vi "RRTPlan.vi"(5 "Parameters.lvclass":refnum<class "Parameters.lvclass">, 6 "Line?":bool, 7 "Volta ao redor\nda área?":bool, 8 "Initial Pos x,y":dbl[](array[numeric]), 9 "Dest x,y":dbl[](array[numeric]), 10 "IA State":T1={"our_robots"=[], "enemy_robots"=[], "balls"=[], "geometry"={"line_width"=0, "field_length"=0, "field_width"=0, "boundary_width"=0, "referee_width"=0, "goal_width"=0, "goal_depth"=0, "goal_wall_width"=0, "center_circle_radius"=0, "defense_radius"=0, "defense_stretch"=0, "free_kick_from_defense_dist"=0, "penalty_spot_from_field_line_dist"=0, "penalty_line_from_spot_dist"=0}, "IA Judge"={"stage"="", "command"="", "our_goalie_id"=0.0, "enemy_goalie_id"=0.0, "command enum"=enum."Halt", "Time"=enum."Azul"}, "Received Timestamp"=timestamp(0 s since 1904-01-01), "Events"={"Touch"=FALSE, "Ball out"=FALSE, "id touch"=0.0, "Ball out of \nVision"=FALSE, "Ball inside \nGoalie area"=FALSE, "Robot not responding"=FALSE, "Robots responding status"=[1.0, 1.0, 1.0, 1.0, 1.0, 1.0], "Enemy Ball \nPossession"=FALSE, "Pass State"=FALSE, "id end of pass"=0.0, "Kick"=FALSE, "Id ini Possession"=0.0, "Ball Possesion"=FALSE, "Id Possesion"=0.0, "Direct Kick"=FALSE, "2nd Strk Ativo"=FALSE}}, 11 "Robot":T2={"id"=0, "function"=enum."Attacker", "x"=0.0, "y"=0.0, "orientation"=0.0, "v_tangent"=0.0, "v_normal"=0.0, "v_ang"=0.0, "kick_x"=0.0, "kick_z"=0.0, "dribble"=FALSE, "Timestamp"=timestamp(0 s since 1904-01-01), "estimatives"={"est_v_tangent"=0.0, "est_v_normal"=0.0, "est_vx"=0.0, "est_vy"=0.0, "Pos Robot Est"=[]}, "dest_x_kick"=0.0, "dest_y_kick"=0.0, "Gap Coord"=[], "States"=enum."GoToTangent", "Path "=[], "Path  Smooth"=[], "Dest"=[], "vx_desired"=0.0, "vy_desired"=0.0, "slowBehavior"=FALSE, "VSSStates"=enum."Pass"}) -> (0 "Path":dbl[][](array[numeric]), 1 "Smooth Path":dbl[][](array[numeric]))   [LabVIEW 2020]
uses:
  Vision_class/Old vision/Controls/AI Robot.ctl
  Vision_class/Old vision/Controls/Functions Enum.ctl
  Vision_class/Old vision/Controls/AttackerStates.ctl
  Vision_class/Old vision/Controls/PathDests.ctl
  Vision_class/Old vision/Controls/PathDest.ctl
  Navigation/VSSNavigation/VSSAttackerStates.ctl
  Vision_class/Old vision/SSL Detection Frame Simple Estimator Cameras VelCmd Folder/Core/AI Input.ctl
  Vision_class/Old vision/SSL Detection Frame Simple Estimator Cameras VelCmd Folder/Core/AI Ball.ctl
  Vision_class/Old vision/SSL Detection Frame Simple Estimator Cameras VelCmd Folder/Core/Field Size.ctl
  Vision_class/Old vision/SSL Detection Frame Simple Estimator Cameras VelCmd Folder/Core/AI Judge.ctl
  Communication_class/Paths/MessageAI_State Folder/Intel/Command Enum.ctl
  Vision_class/Old vision/SSL Detection Frame Simple Estimator Cameras VelCmd Folder/Util/Events/Events.ctl
  Parameters_class/Parameters.lvclass
  Utilities_class/Utilities.lvclass
  Parameters_class/Parameters.lvclass/Parameters.ctl
  <vilib>/Analysis/_algsub.llb/Real Vector Norm.vi
  Parameters_class/Read Project.vi
  <vilib>/Analysis/NI_AALPro.lvlib
panel:
  in  "Path out":dbl[][](array[numeric])
  out "Path out 2":dbl[][](array[numeric])
  in  "WayPointProb":dbl=0.6 format="%#_13g"
  in  "GoalProb":dbl=0.1 format="%#_13g"
  in  "Step":dbl=80.0
  out "Goal":dbl[](array[numeric])
  out "Initial State":dbl[](array[numeric])
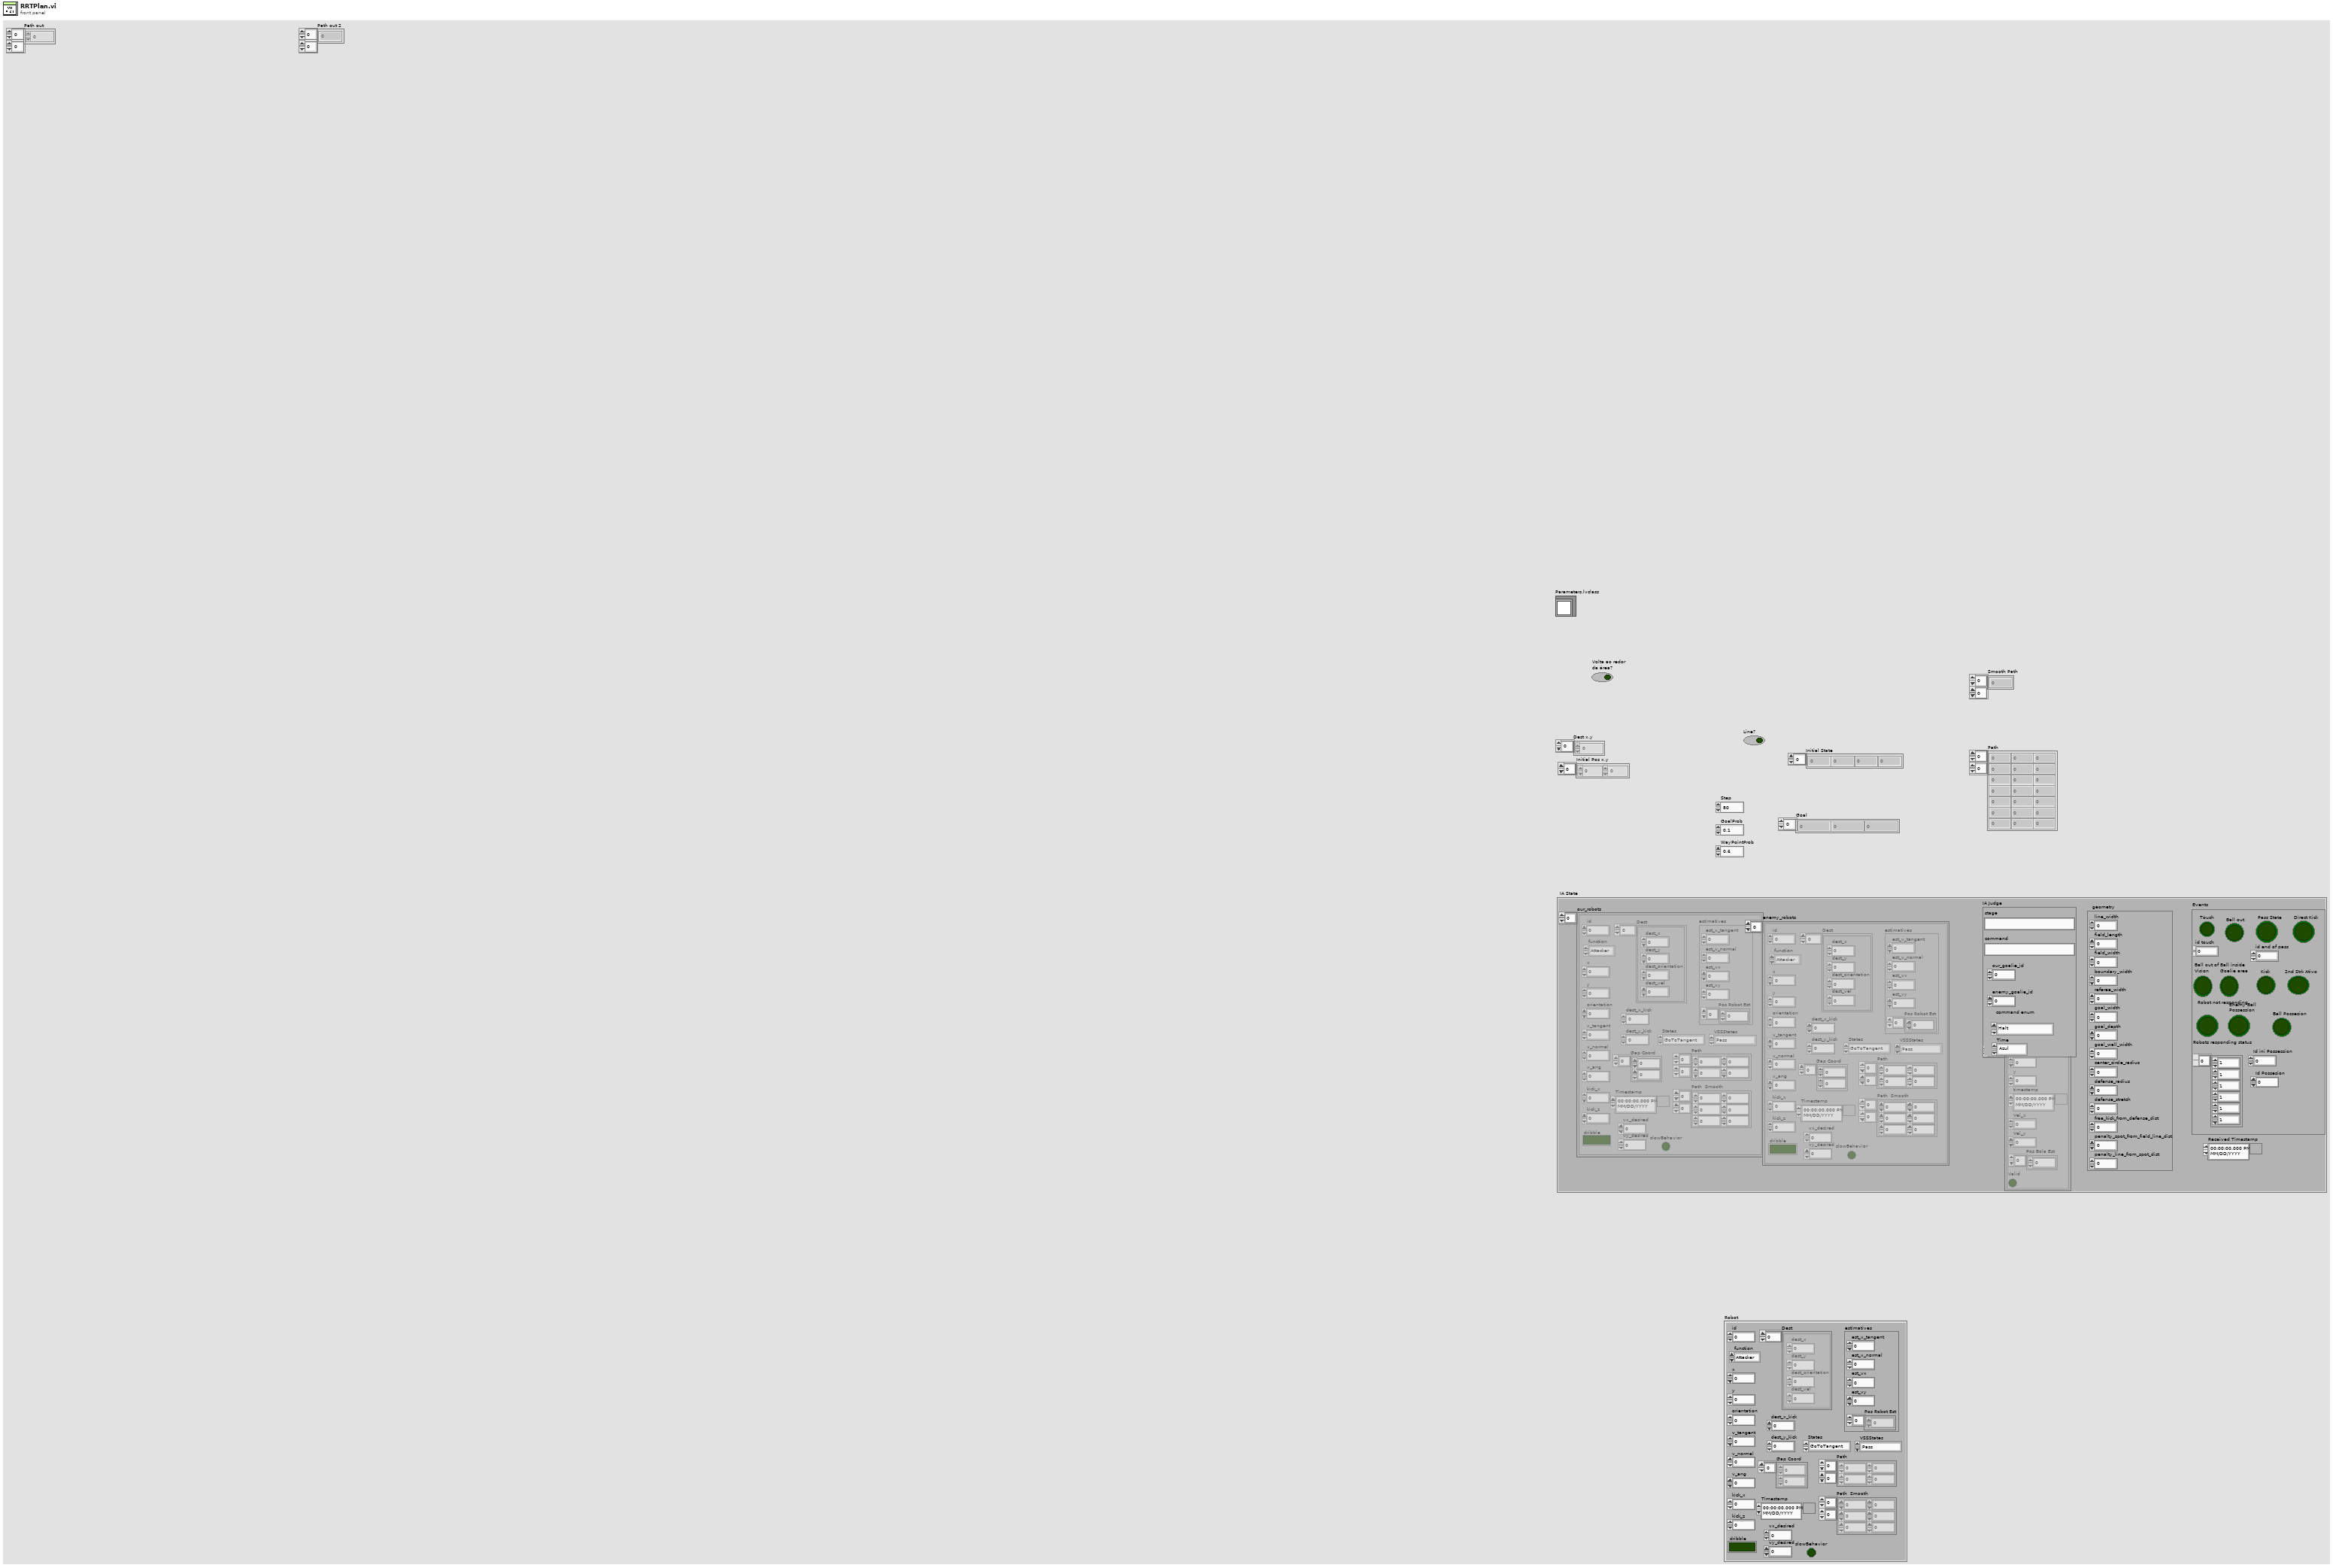
[diagram p1: front panel]
types:
  T1 = typedef "AI Input.ctl" = cluster{"our_robots":T2[], "enemy_robots":T2[], "balls":T8[], "geometry":T9, "IA Judge":T10, "Received Timestamp":timestamp, "Events":T12}
  T2 = typedef "AI Robot.ctl" = cluster{"id":u32, "function":T3, "x":dbl, "y":dbl, "orientation":dbl, "v_tangent":dbl, "v_normal":dbl, "v_ang":dbl, "kick_x":dbl, "kick_z":dbl, "dribble":bool, "Timestamp":timestamp, "estimatives":cluster{"est_v_tangent":dbl, "est_v_normal":dbl, "est_vx":dbl, "est_vy":dbl, "Pos Robot Est":dbl[]}, "dest_x_kick":dbl, "dest_y_kick":dbl, "Gap Coord":dbl[], "States":T4, "Path ":dbl[][], "Path  Smooth":dbl[][], "Dest":T5, "vx_desired":dbl, "vy_desired":dbl, "slowBehavior":bool, "VSSStates":T7}
  T3 = typedef "Functions Enum.ctl" = enum16{"2nd Striker", "Attacker", "Goalie", "Defender", "Striker", "Goto 0", "Dummy", "Kicker", "ZigZag 0", "ZigZag 1", "ZigZag 2", "ZigZag 3", "ZigZag 4", "ZigZag 5", "ZigZag 6", "ZigZag 7", "ZigZag 8", ""}
  T4 = typedef "AttackerStates.ctl" = enum16{"Pass", "GoToTangent", "BallGetting", "GoToKick", ""}
  T5 = typedef "PathDests.ctl" = T6[]
  T6 = typedef "PathDest.ctl" = cluster{"dest_x":dbl, "dest_y":dbl, "dest_orientation":dbl, "dest_vel":dbl}
  T7 = typedef "VSSAttackerStates.ctl" = enum16{"Pass", "GoToTangent", "BallGetting", "GoToKick", "Rotate anti-clockwise", "Rotate Clockwise", ""}
  T8 = typedef "AI Ball.ctl" = cluster{"x":dbl, "y":dbl, "timestamp":timestamp, "Vel_x":dbl, "Vel_y":dbl, "Pos Bola Est":dbl[], "Valid":bool}
  T9 = typedef "Field Size.ctl" = cluster{"line_width":u32, "field_length":u32, "field_width":u32, "boundary_width":u32, "referee_width":u32, "goal_width":u32, "goal_depth":u32, "goal_wall_width":u32, "center_circle_radius":u32, "defense_radius":u32, "defense_stretch":u32, "free_kick_from_defense_dist":u32, "penalty_spot_from_field_line_dist":u32, "penalty_line_from_spot_dist":u32}
  T10 = typedef "AI Judge.ctl" = cluster{"stage":string, "command":string, "our_goalie_id":dbl, "enemy_goalie_id":dbl, "command enum":T11, "Time":enum16{"Azul", "Amarelo"}}
  T11 = typedef "Command Enum.ctl" = enum16{"Halt", "Stop", "Force Start", "PKA Normal Start", "Prepare Kickoff Ally", "PKE Normal Start", "Prepare Kickoff Enemy", "Prepare Penalty Ally", "PPA Normal Start", "Prepare Penalty Enemy", "PPE Normal Start", "Direct Free Enemy", "Direct Free Ally", "Indirect Free Enemy", "Indirect Free Ally", "Timeout Enemy", "Timeout Ally", "Goal Enemy", "Goal Ally", "Ball Placement Enemy", "Ball Placement Ally", "Normal Half Time", "Extra Time Break", "Extra Half Time", "None", "Post Game"}
  T12 = typedef "Events.ctl" = cluster{"Touch":bool, "Ball out":bool, "id touch":dbl, "Ball out of \nVision":bool, "Ball inside \nGoalie area":bool, "Robot not responding":bool, "Robots responding status":dbl[], "Enemy Ball \nPossession":bool, "Pass State":bool, "id end of pass":dbl, "Kick":bool, "Id ini Possession":dbl, "Ball Possesion":bool, "Id Possesion":dbl, "Direct Kick":bool, "2nd Strk Ativo":bool}
  T13 = typedef "Project.ctl" = enum16{"SSL", "VSS"}
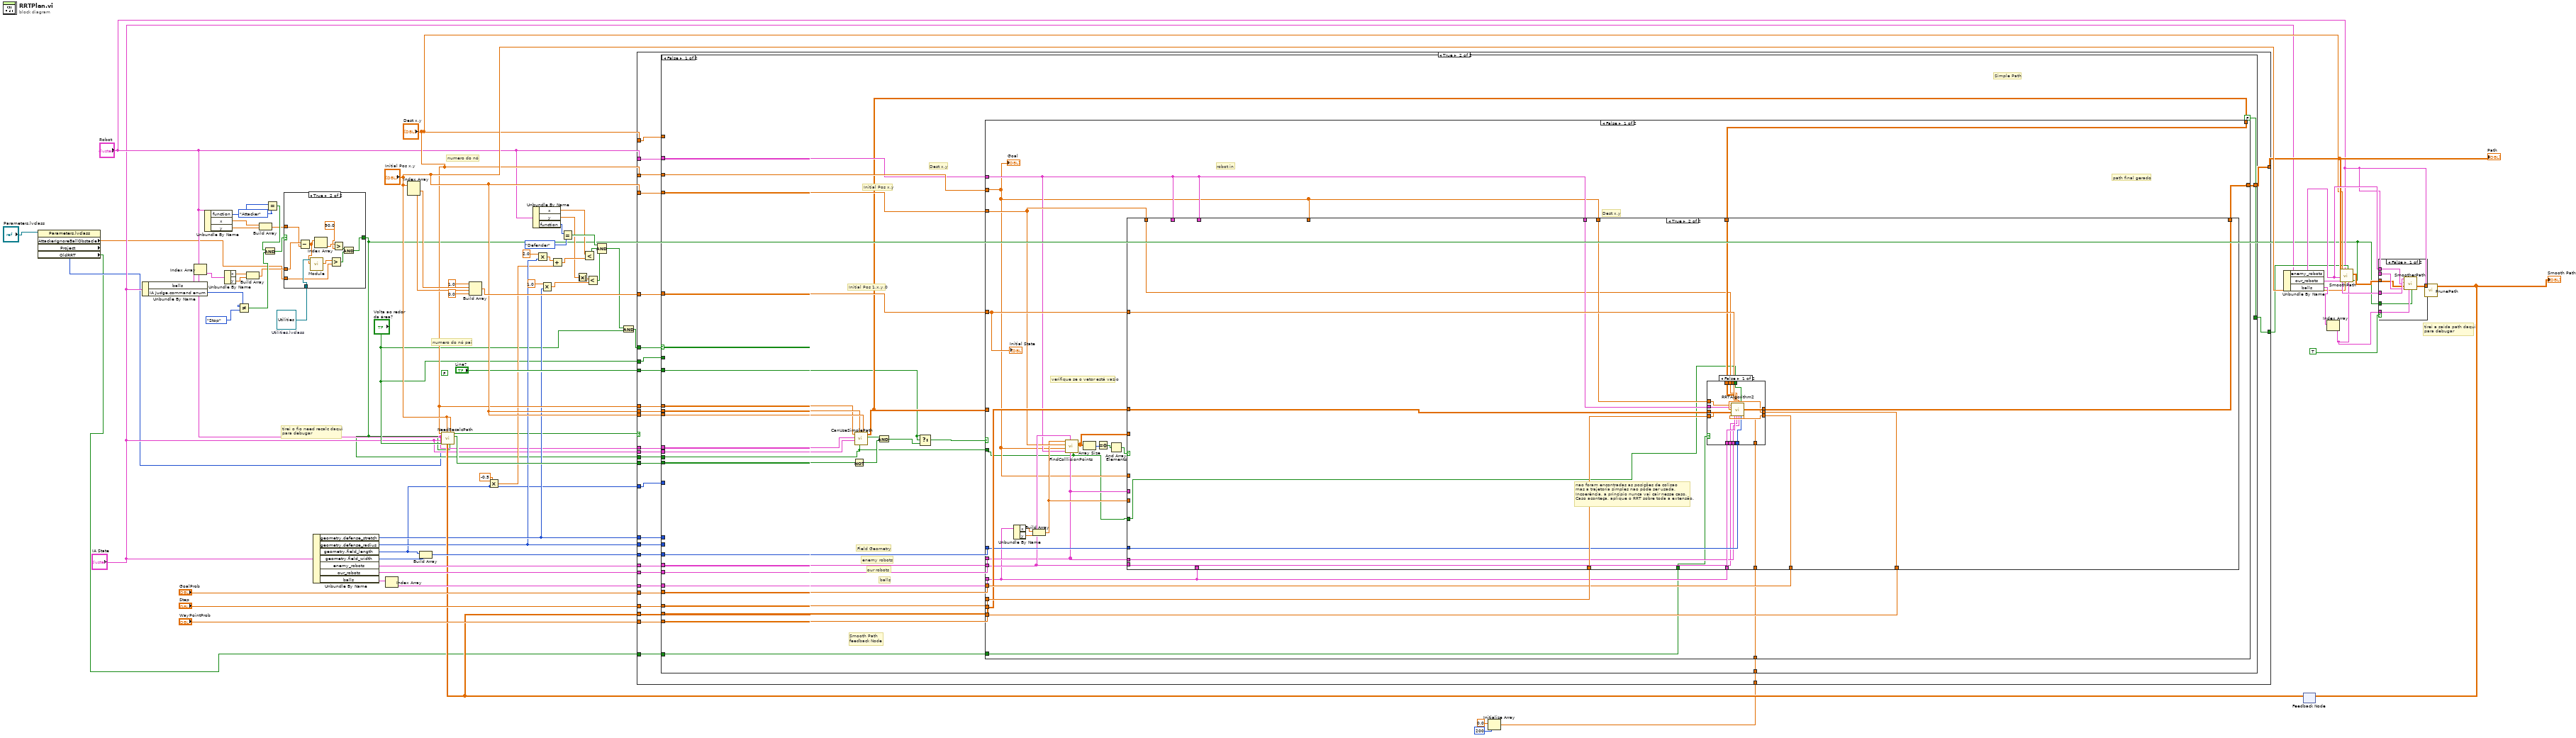
[diagram p0: block diagram]
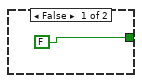
[diagram p2: hidden frame]
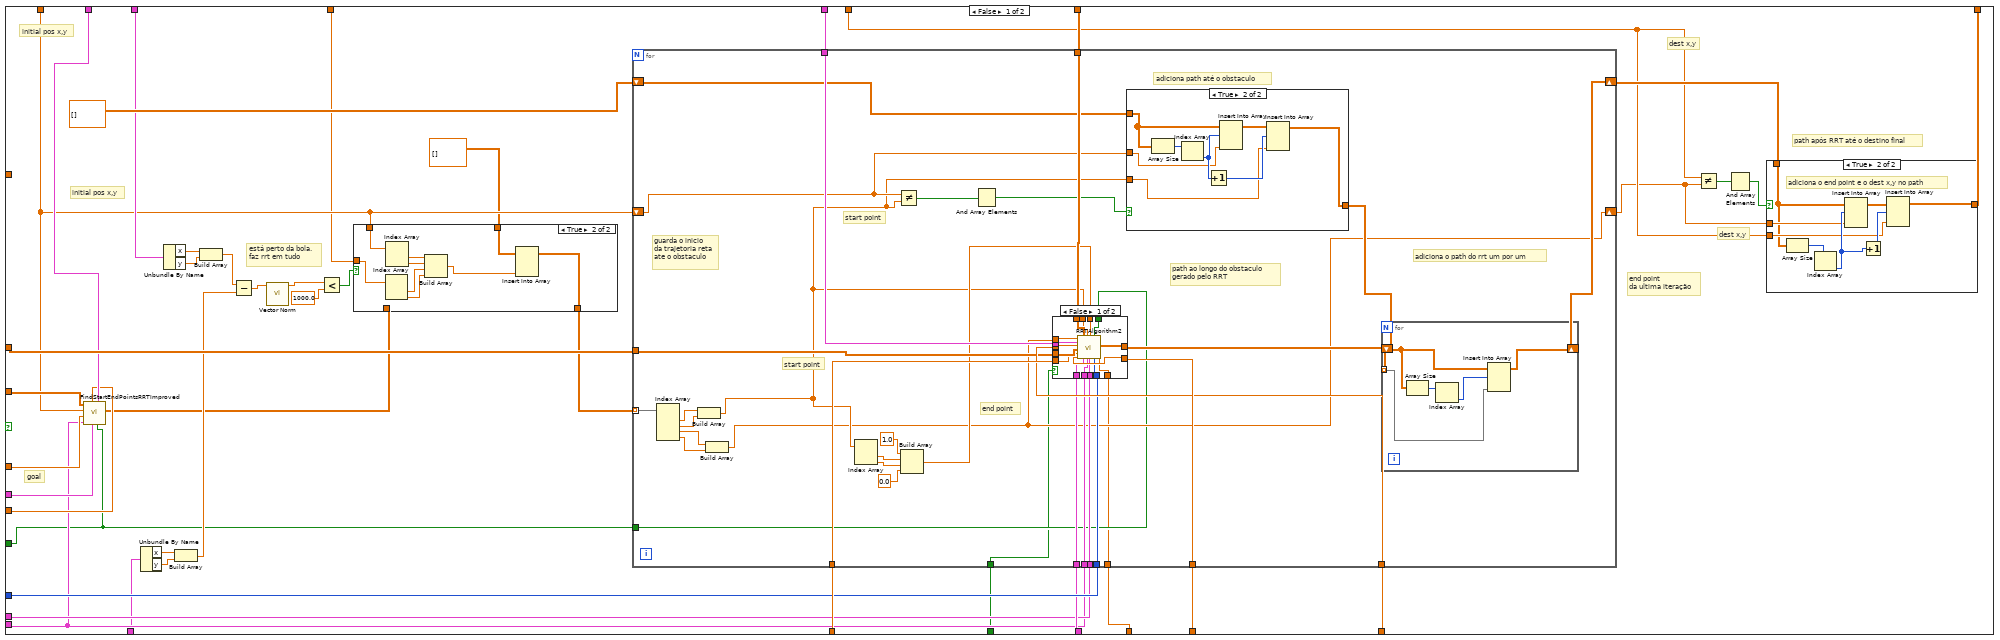
[diagram p4: hidden frame]
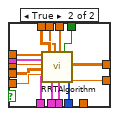
[diagram p7: hidden frame]
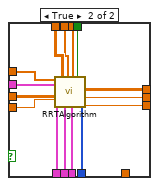
[diagram p9: hidden frame]
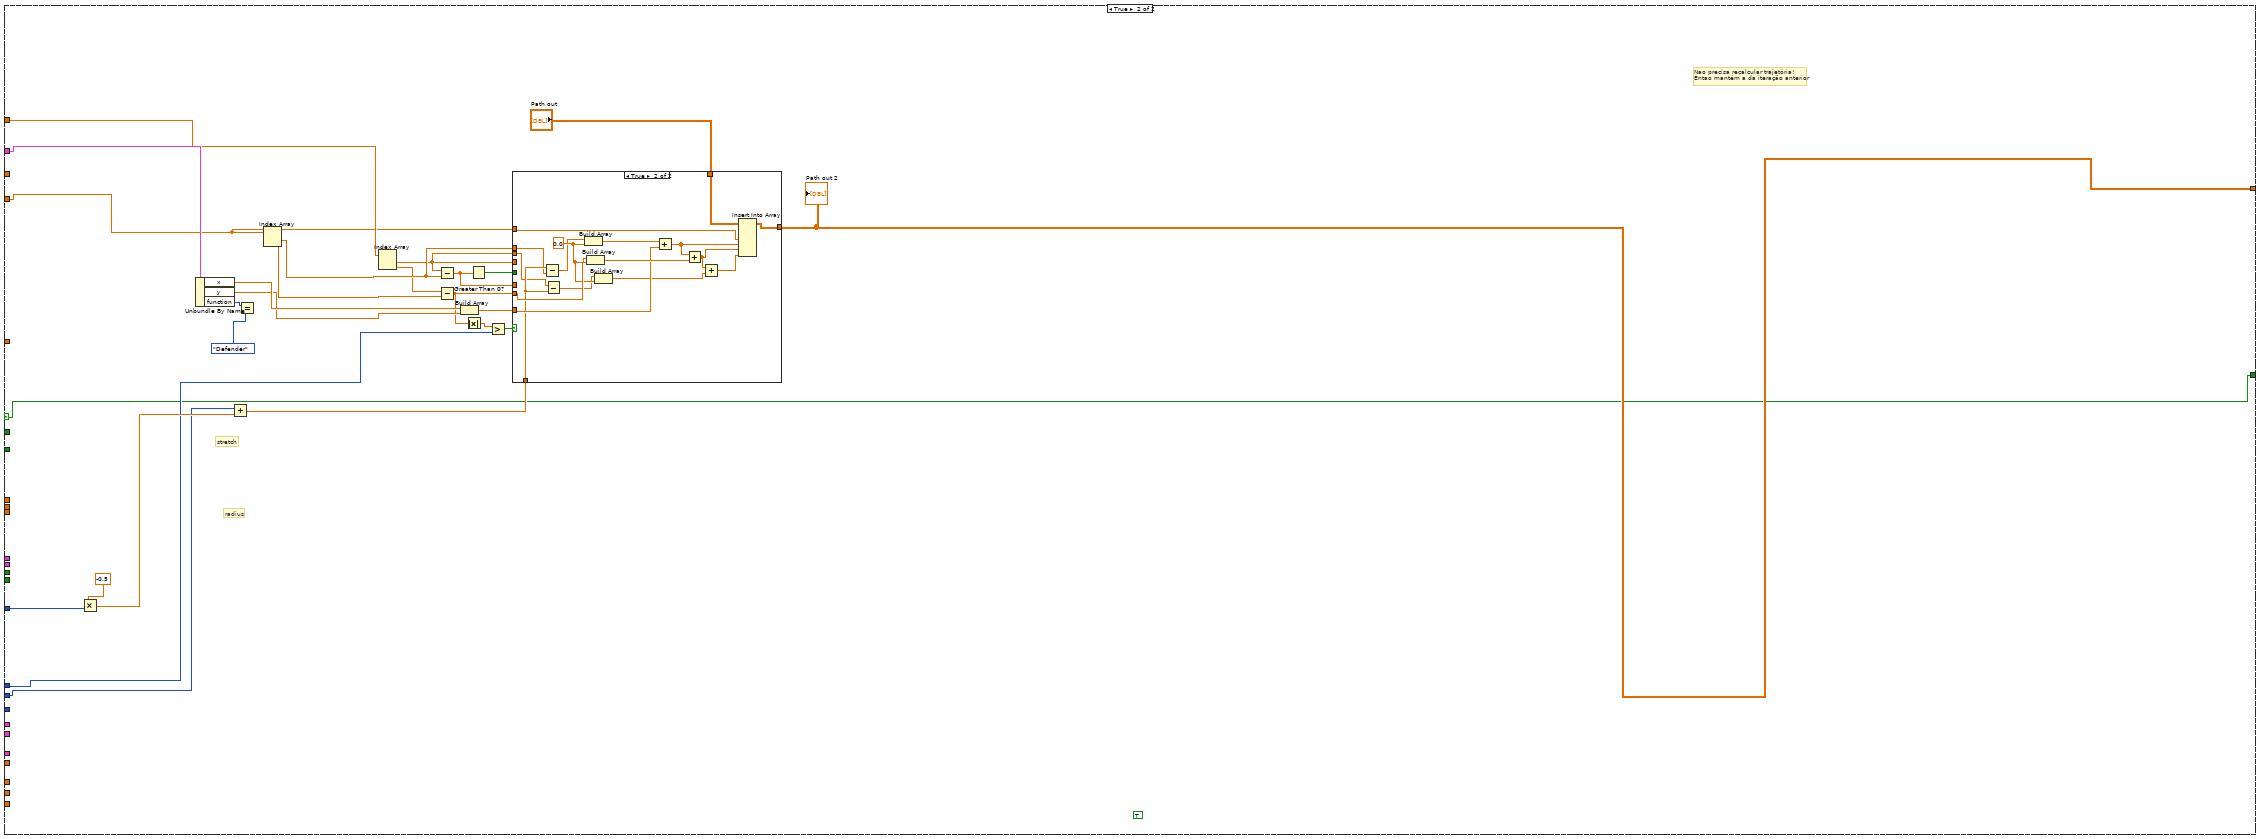
[diagram p11: hidden frame]
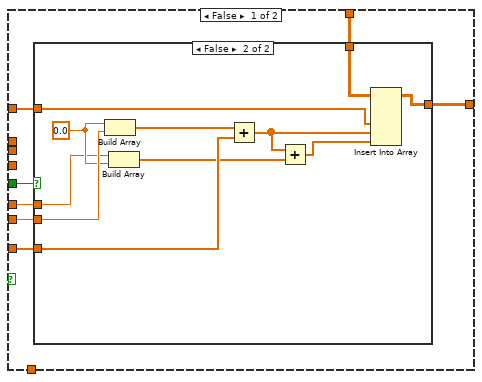
[diagram p12: hidden frame]
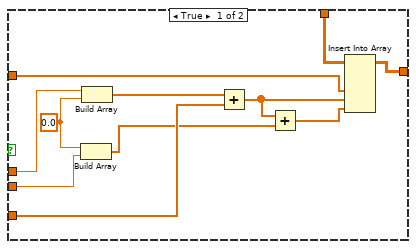
[diagram p13: hidden frame]
diagram:
  w10 = refnum<class "Utilities.lvclass"> refnum  # Utilities.lvclass
  (unwired) FALSE
  # "tirei a saida path daqui\npara debugar"
  # "tirei o fio need recalc daqui\npara debugar"
  # "numero do nó pai"
  # "numero do nó"
  n1 = property class="Parameters.lvclass"(reference="Parameters.lvclass") -> ("AttackerIgnoreBallObstacle"=w8:dbl, "Project"=w5:T13, "OldRRT"=w1:bool)  [unwired: 1 in, 2 out]
  n2 = Unbundle By Name("IA State") -> ("balls"=w23:T8[], "IA Judge.command enum"=w16:T11)
  n3 = Index Array(array=w23) -> (element=w22:T8)  [unwired: 1 in]
  n4 = Unbundle By Name("Robot") -> ("function"=w19:T3, "x"=w26:dbl, "y"=w25:dbl)
  n5 = Unbundle By Name(w22) -> ("x"=w21:dbl, "y"=w20:dbl)
  n6 = Not Equal?(x=w16, y=Command_Enum."Stop" ("IA Judge.command enum")) -> (x != y?=w14:bool)
  n7 = Build Array(w21, w20) -> (w11:dbl[])
  n8 = Build Array(w26, w25) -> (w12:dbl[])
  n9 = Equal?(x=w19, y=Functions_Enum."Attacker" ("function")) -> (x = y?=w13:bool)
  n10 = And(x=w13, y=w14) -> (x .and. y?=w17:bool)
  n11 = case shown="True" w17 {
    tunnel: w12 -> [_ w88]
    tunnel: w11 -> [_ w89]
    tunnel: [FALSE w83] -> w6
    tunnel: w10 -> [_ w87]
    tunnel: w8 -> [_ w82]
    frame False {
    }
    frame True {
      n12 = Subtract(x=w89, y=w88) -> (x-y=w86:dbl[])
      n13 = call-dynamic "Module.vi"("2D vector"=w86, "Utilities in"=w87) -> ("Modulo"=w85:dbl)  [unwired: 7 in, 2 out]
      n14 = Index Array(array=w86) -> (element=w81:dbl)  [unwired: 1 in]
      n15 = Greater?(x=w85, y=w82) -> (0:w84:bool)
      n16 = Greater?(x=w81, y=90.0) -> (0:w79:bool)
      n17 = And(x=w79, y=w84) -> (x .and. y?=w83:bool)
    }
  }
  n18 = Unbundle By Name("IA State") -> ("geometry.defense_stretch"=w35:u32, "geometry.defense_radius"=w34:u32, "geometry.field_length"=w32:u32, "geometry.field_width"=w50:u32, "enemy_robots"=w73:T2[], "our_robots"=w70:T2[], "balls"=w66:T8[])
  n19 = Index Array(array=w66) -> (element=w65:T8)  [unwired: 1 in]
  n20 = Index Array(array="Initial Pos x,y") -> (element #1=w69:dbl, element #2=w68:dbl)  [unwired: 2 in]
  n21 = Build Array(w32, w50) -> (w77:u32[])
  n22 = Build Array(1.0 ("element"), w69, w68, 0.0 ("element")) -> (w63:dbl[])
  n23 = Multiply(x=-0.5, y=w32) -> (x*y=w31:dbl)
  n24 = Unbundle By Name("Robot") -> ("x"=w37:dbl, "y"=w36:dbl, "function"=w48:T3)
  n25 = Multiply(x=2.0, y=w34) -> (x*y=w45:dbl)
  n26 = Multiply(x=1.0, y=w35) -> (x*y=w39:dbl)
  n27 = Add(x=w45, y=w31) -> (x+y=w44:dbl)
  n28 = Equal?(x=w48, y=Functions_Enum."Defender") -> (x = y?=w42:bool)
  n29 = Absolute Value(x=w36) -> (abs(x)=w41:dbl)
  n30 = Less?(x=w37, y=w44) -> (x < y?=w43:bool)
  n31 = Less?(x=w41, y=w39) -> (x < y?=w38:bool)
  n32 = Compound Arithmetic op=AND(w42, w43, w38) -> (w30:bool)
  n33 = And(x=w30, y="Volta ao redor\nda área?") -> (x .and. y?=w28:bool)
  n34 = Initialize Array(0.0 ("element"), 200 ("dimension size")) -> (w2:dbl[])
  n35 = Unbundle By Name("IA State") -> ("enemy_robots"=w59:T2[], "our_robots"=w60:T2[], "balls"=w67:T8[])
  n36 = feedback #1() -> (w64:dbl[][])  [unwired: 1 in]
  n37 = call "NeedRecalcPath.vi"("Project"=w5, "ignoreBall?"=w6, "Initial State"="Initial Pos x,y", "SmoothPath"=w64, "Pos x,y"="Initial Pos x,y", "Volta ao redor\nda área?"="Volta ao redor\nda área?", "IA State"="IA State", "Robot"="Robot", "Dest x,y"="Dest x,y") -> ("result"=w62:bool, "NeedRecalc"=w7:bool)  [unwired: 1 in]
  n38 = case shown="True" w7 {
    tunnel: w77 -> [_ w121]
    tunnel: "Step" -> [_ w120]
    tunnel: "GoalProb" -> [_ w119]
    tunnel: "WayPointProb" -> [_ w118]
    tunnel: w73 -> [_ w117]
    tunnel: w63 -> [_ w116]
    tunnel: w64 -> [w91 w115]
    tunnel: w70 -> [_ w114]
    tunnel: [w91 w113] -> w54
    tunnel: "Dest x,y" -> [_ w112]
    tunnel: "Initial Pos x,y" -> [_ w111]
    tunnel: "Robot" -> [_ w110]
    tunnel: w65 -> [_ w109]
    tunnel: "Initial Pos x,y" -> [_ w108]
    tunnel: "Initial Pos x,y" -> [_ w107]
    tunnel: "Dest x,y" -> [_ w106]
    tunnel: "Robot" -> [_ w105]
    tunnel: "IA State" -> [_ w104]
    tunnel: w62 -> [_ w103]
    tunnel: w35 -> [_ w99]
    tunnel: w34 -> [_ w98]
    tunnel: "Dest x,y" -> [_ w95]
    tunnel: w32 -> [_ w97]
    tunnel: [w90 w102] -> w51
    tunnel: "Line?" -> [_ w101]
    tunnel: "Volta ao redor\nda área?" -> [_ w96]
    tunnel: w28 -> [w90 w100]
    tunnel: w6 -> [_ w94]
    tunnel: w1 -> [_ w93]
    tunnel: w2 -> [_ w92]
    frame False {
    }
    frame True {
      n39 = case shown="False" w100 {
        selector: w100 -> [_ w362]
        tunnel: w121 -> [w150 _]
        tunnel: w120 -> [w149 _]
        tunnel: w119 -> [w148 _]
        tunnel: w118 -> [w147 _]
        tunnel: w117 -> [w146 _]
        tunnel: w116 -> [w145 _]
        tunnel: w115 -> [w144 _]
        tunnel: w114 -> [w143 _]
        tunnel: [w142 w372] -> w113
        tunnel: w112 -> [w141 _]
        tunnel: w111 -> [w140 w373]
        tunnel: w110 -> [w139 w375]
        tunnel: w109 -> [w138 _]
        tunnel: w108 -> [w137 _]
        tunnel: w107 -> [w136 _]
        tunnel: w106 -> [w135 _]
        tunnel: w105 -> [w134 _]
        tunnel: w104 -> [w133 _]
        tunnel: w103 -> [w131 _]
        tunnel: [FALSE w362] -> w102
        tunnel: w101 -> [w126 _]
        tunnel: w99 -> [_ w378]
        tunnel: w98 -> [_ w377]
        tunnel: w97 -> [_ w376]
        tunnel: w96 -> [_ _]
        tunnel: w95 -> [_ w374]
        tunnel: w94 -> [w124 _]
        tunnel: w93 -> [w123 _]
        tunnel: w92 -> [w122 _]
        frame False {
          # "Initial Pos 1,x,y,0"
          # "Initial Pos x,y"
          # "Dest x,y"
          # "Simple Path"
          # "balls"
          # "our robots"
          # "enemy robots"
          # "Field Geometry"
          # "Smooth Path \nfeedback Node"
          n40 = Not(x=w131) -> (.not. x?=w130:bool)
          n41 = call "CanUseSimplePath.vi"("Initial State"=w137, "ignoreBall?"=w124, "Pos x,y"=w136, "IA State"=w133, "Robot"=w134, "Dest x,y"=w135) -> (2:"Simple Path"=w132:bool, 3:"Simple Path"=w129:dbl[][])  [unwired: 4 in]
          n42 = And(x=w132, y=w130) -> (x .and. y?=w127:bool)
          n43 = Select(t=w126, s=w126, f=w127) -> (s? t:f=w128:bool)
          n44 = case shown="False" w128 {
            tunnel: w150 -> [w170 _]
            tunnel: w149 -> [w174 _]
            tunnel: w139 -> [w156 _]
            tunnel: w148 -> [w173 _]
            tunnel: w147 -> [w172 _]
            tunnel: w146 -> [w157 _]
            tunnel: w144 -> [w171 _]
            tunnel: [w167 w361] -> w142
            tunnel: w141 -> [w154 _]
            tunnel: w140 -> [w159 _]
            tunnel: w145 -> [w169 _]
            tunnel: w143 -> [w164 _]
            tunnel: w138 -> [w155 _]
            tunnel: w129 -> [_ w361]
            tunnel: w129 -> [w168 _]
            tunnel: w124 -> [w153 _]
            tunnel: w123 -> [w152 _]
            tunnel: w122 -> [w151 _]
            frame False {
              # "robot in"
              # "path final gerado"
              # "Dest x,y"
              # "verifique se o vetor está vazio"
              n45 = Unbundle By Name(w155) -> ("x"=w166:dbl, "y"=w165:dbl)
              n46 = Build Array(w166, w165) -> (w158:dbl[])
              n47 = call "FindColllisionPoints.vi"("ignoreBall?"=w153, "enemy_robots"=w157, "our_robots"=w164, "Robot in"=w156, "Goal"=w154, "Initial State"=w159, "ball"=w158) -> ("Collision Points"=w160:dbl[][])  [unwired: 4 in]
              n48 = Array Size(array=w160) -> (size(s)=w163:i32[])
              n49 = Equal To 0?(x=w163) -> (x = 0?=w161:bool[])
              n50 = And Array Elements(Boolean array=w161) -> (logical AND=w162:bool)
              n51 = case shown="True" w162 {
                tunnel: w174 -> [w216 w329]
                tunnel: w173 -> [w215 w328]
                tunnel: w172 -> [w214 w327]
                tunnel: w171 -> [w213 w326]
                tunnel: w170 -> [w212 w325]
                tunnel: w169 -> [_ w324]
                tunnel: w168 -> [w211 w323]
                tunnel: [w201 w322] -> w167
                tunnel: w155 -> [w210 w321]
                tunnel: w154 -> [w200 w320]
                tunnel: w156 -> [w209 w319]
                tunnel: w157 -> [w208 w318]
                tunnel: w164 -> [w195 w317]
                tunnel: w160 -> [w207 _]
                tunnel: w159 -> [w180 w316]
                tunnel: w154 -> [w206 _]
                tunnel: w156 -> [w198 _]
                tunnel: w158 -> [w197 _]
                tunnel: w157 -> [w196 _]
                tunnel: w156 -> [w194 _]
                tunnel: w155 -> [w193 _]
                tunnel: w154 -> [w179 _]
                tunnel: w153 -> [w177 w315]
                tunnel: w152 -> [w176 w313]
                tunnel: w151 -> [w175 w314]
                frame False {
                  # "está perto da bola.\nfaz rrt em tudo"
                  # "dest x,y"
                  # "end point \nda ultima iteração"
                  # "dest x,y"
                  # "path após RRT até o destino final"
                  # "initial pos x,y"
                  # "initial pos x,y"
                  # "goal"
                  n52 = call "FindStartEndPointsRRTImproved.vi"("ignoreBall?"=w177, "Robot in"=w198, "enemy_robots"=w196, "ball"=w197, "our_robots"=w195, "Goal"=w206, "Initial State"=w180, "Collision Points"=w207) -> ("Start End Points RRT"=w182:dbl[][])  [unwired: 3 in]
                  n53 = Unbundle By Name(w193) -> ("x"=w190:dbl, "y"=w189:dbl)
                  n54 = Unbundle By Name(w194) -> ("x"=w192:dbl, "y"=w191:dbl)
                  n55 = Build Array(w190, w189) -> (w187:dbl[])
                  n56 = Build Array(w192, w191) -> (w188:dbl[])
                  n57 = Subtract(x=w188, y=w187) -> (x-y=w186:dbl[])
                  n58 = call-poly <vilib>:"Vector Norm.vi"("Input Vector"=w186) -> ("norm"=w185:dbl)  [unwired: 9 in, 1 out]
                  n59 = Less?(x=w185, y=1000.0) -> (x < y?=w183:bool)
                  n60 = case shown="True" w183 {
                    tunnel: [w217 w218] -> w181
                    tunnel: w182 -> [w217 _]
                    tunnel: w180 -> [_ w226]
                    tunnel: w179 -> [_ w223]
                    tunnel: dbl[][] [] -> [_ w220]
                    frame False {
                    }
                    frame True {
                      n61 = Index Array(array=w223) -> (element #1=w222:dbl, element #2=w221:dbl)  [unwired: 2 in]
                      n62 = Index Array(array=w226) -> (element #1=w225:dbl, element #2=w224:dbl)  [unwired: 2 in]
                      n63 = Build Array(w225, w224, w222, w221) -> (w219:dbl[])
                      n64 = Insert Into Array(array=w220, new element=w219) -> (w218:dbl[][])  [unwired: 2 in]
                    }
                  }
                  n65 = for {
                    tunnel: w216 -> [w267]
                    tunnel: w215 -> [w266]
                    tunnel: w214 -> [w265]
                    tunnel: w213 -> [w264]
                    tunnel: w212 -> [w263]
                    tunnel: w211 -> [w262]
                    tunnel: w210 -> [w261]
                    tunnel: w209 -> [w260]
                    tunnel: w208 -> [w259]
                    tunnel: w195 -> [w258]
                    tunnel: w181 -> [w248] mode=indexing
                    shift-right: [w239] -> w199
                    shift-left: w180 -> [w242]
                    shift-right: [w240] -> w202
                    shift-left: dbl[][] [] -> [w243]
                    tunnel: w177 -> [w238]
                    tunnel: w176 -> [w237]
                    tunnel: w175 -> [w236]
                    # "adiciona o path do rrt um por um"
                    # "start point"
                    # "guarda o inicio\nda trajetoria reta\nate o obstaculo"
                    # "end point"
                    # "start point"
                    # "path ao longo do obstaculo\ngerado pelo RRT"
                    # "adiciona path até o obstaculo"
                    n66 = Index Array(array=w248) -> (element #1=w247:dbl, element #2=w246:dbl, element #3=w245:dbl, element #4=w244:dbl)  [unwired: 4 in]
                    n67 = Build Array(w247, w246) -> (w241:dbl[])
                    n68 = Build Array(w245, w244) -> (w239:dbl[])
                    n69 = Index Array(array=w241) -> (element #1=w255:dbl, element #2=w254:dbl)  [unwired: 2 in]
                    n70 = Not Equal?(x=w242, y=w241) -> (x != y?=w251:bool[])
                    n71 = Build Array(1.0 ("element"), w255, w254, 0.0 ("element")) -> (w253:dbl[])
                    n72 = And Array Elements(Boolean array=w251) -> (logical AND=w250:bool)
                    n73 = case shown="False" w237 {
                      tunnel: w267 -> [w277 w298]
                      tunnel: w266 -> [w282 w297]
                      tunnel: w265 -> [w279 w296]
                      tunnel: w264 -> [w278 w295]
                      tunnel: w263 -> [w276 w294]
                      tunnel: w262 -> [w272 w293]
                      tunnel: w261 -> [w273 w292]
                      tunnel: w260 -> [w280 w291]
                      tunnel: w259 -> [w275 w290]
                      tunnel: w258 -> [w274 w289]
                      tunnel: w253 -> [w271 w288]
                      tunnel: [w283 w287] -> w252
                      tunnel: w241 -> [w270 w286]
                      tunnel: w239 -> [w281 w285]
                      tunnel: w238 -> [w269 w284]
                      tunnel: w236 -> [w268 _]
                      frame False {
                        n74 = call "RRTAlgorithm2.vi"("Dest x,y"=w281, "Robot"=w280, "WayPointProb"=w279, "Path in \n(Smooth do Feedback Node)"=w278, "Step"=w277, "GoalProb"=w282, "Simple Path"=w272, "Ball"=w273, "Initial Pos x,y"=w270, "our_robots"=w274, "Initial Pos 1,x,y,0"=w271, "enemy_robots"=w275, "ignoreBall?"=w269, "Field Geomtery"=w276, "buffer"=w268) -> ("Path"=w283:dbl[][])  [unwired: 4 in]
                      }
                      frame True {
                        n75 = call "RRTAlgorithm.vi"("Dest x,y"=w285, "Robot"=w291, "WayPointProb"=w296, "Path in \n(Smooth do Feedback Node)"=w295, "Step"=w298, "GoalProb"=w297, "Simple Path"=w293, "Ball"=w292, "Initial Pos x,y"=w286, "our_robots"=w289, "Initial Pos 1,x,y,0"=w288, "enemy_robots"=w290, "ignoreBall?"=w284, "Field Geomtery"=w294) -> ("Path"=w287:dbl[][])  [unwired: 5 in]
                      }
                    }
                    n76 = case shown="True" w250 {
                      tunnel: [w299 w304] -> w249
                      tunnel: w243 -> [w299 w306]
                      tunnel: w242 -> [_ w301]
                      tunnel: w241 -> [_ w300]
                      frame False {
                      }
                      frame True {
                        n77 = Array Size(array=w306) -> (size(s)=w307:i32[])
                        n78 = Index Array(array=w307) -> (element=w303:i32)  [unwired: 1 in]
                        n79 = Increment(x=w303) -> (x+1=w302:i32)
                        n80 = Insert Into Array(array=w306, index (row)=w303, new element=w301) -> (w305:dbl[][])  [unwired: 1 in]
                        n81 = Insert Into Array(array=w305, index (row)=w302, new element=w300) -> (w304:dbl[][])  [unwired: 1 in]
                      }
                    }
                    n82 = for {
                      tunnel: w252 -> [w311] mode=indexing
                      shift-right: [w310] -> w240
                      shift-left: w249 -> [w312]
                      n83 = Array Size(array=w312) -> (size(s)=w309:i32[])
                      n84 = Index Array(array=w309) -> (element=w308:i32)  [unwired: 1 in]
                      n85 = Insert Into Array(array=w312, index (row)=w308, new element=w311) -> (w310:dbl[][])  [unwired: 1 in]
                    }
                  }
                  n86 = Not Equal?(x=w200, y=w199) -> (x != y?=w204:bool[])
                  n87 = And Array Elements(Boolean array=w204) -> (logical AND=w203:bool)
                  n88 = case shown="True" w203 {
                    tunnel: [w227 w229] -> w201
                    tunnel: w200 -> [_ w231]
                    tunnel: w199 -> [_ w230]
                    tunnel: w202 -> [w227 w228]
                    frame False {
                    }
                    frame True {
                      # "adiciona o end point e o dest x,y no path"
                      n89 = Array Size(array=w228) -> (size(s)=w235:i32[])
                      n90 = Index Array(array=w235) -> (element=w233:i32)  [unwired: 1 in]
                      n91 = Insert Into Array(array=w228, index (row)=w233, new element=w230) -> (w234:dbl[][])  [unwired: 1 in]
                      n92 = Increment(x=w233) -> (x+1=w232:i32)
                      n93 = Insert Into Array(array=w234, index (row)=w232, new element=w231) -> (w229:dbl[][])  [unwired: 1 in]
                    }
                  }
                }
                frame True {
                  # "nao foram encontradas as posições de colisao\nmas a trajetoria simples nao pôde ser usada.\nIncoerência, a princípio nunca vai cair nesse caso.\nCaso aconteça, aplique o RRT sobre toda a extensão."
                  n94 = case shown="False" w313 {
                    tunnel: w329 -> [w331 w360]
                    tunnel: w328 -> [w344 w359]
                    tunnel: w327 -> [w343 w358]
                    tunnel: w326 -> [w332 w357]
                    tunnel: w325 -> [w338 w356]
                    tunnel: w324 -> [w341 w355]
                    tunnel: w323 -> [w339 w354]
                    tunnel: [w345 w353] -> w322
                    tunnel: w321 -> [w337 w352]
                    tunnel: w320 -> [w334 w351]
                    tunnel: w319 -> [w333 w350]
                    tunnel: w318 -> [w335 w349]
                    tunnel: w317 -> [w336 w348]
                    tunnel: w316 -> [w340 w347]
                    tunnel: w315 -> [w342 w346]
                    tunnel: w314 -> [w330 _]
                    frame False {
                      n95 = call "RRTAlgorithm2.vi"("Dest x,y"=w334, "Robot"=w333, "WayPointProb"=w343, "Path in \n(Smooth do Feedback Node)"=w332, "Step"=w331, "GoalProb"=w344, "Simple Path"=w339, "Ball"=w337, "Initial Pos x,y"=w340, "our_robots"=w336, "Initial Pos 1,x,y,0"=w341, "enemy_robots"=w335, "ignoreBall?"=w342, "Field Geomtery"=w338, "buffer"=w330) -> ("Path"=w345:dbl[][])  [unwired: 4 in]
                    }
                    frame True {
                      n96 = call "RRTAlgorithm.vi"("Dest x,y"=w351, "Robot"=w350, "WayPointProb"=w358, "Path in \n(Smooth do Feedback Node)"=w357, "Step"=w360, "GoalProb"=w359, "Simple Path"=w354, "Ball"=w352, "Initial Pos x,y"=w347, "our_robots"=w348, "Initial Pos 1,x,y,0"=w355, "enemy_robots"=w349, "ignoreBall?"=w346, "Field Geomtery"=w356) -> ("Path"=w353:dbl[][])  [unwired: 5 in]
                    }
                  }
                }
              }
              "Initial State" <- w169
              "Goal" <- w154
            }
            frame True {
              # "Pode usar a trajetória simples (reta) entre o estado inicial e o destino.\nAlém disso, nao precisa recalcular a trajetória."
            }
          }
        }
        frame True {
          (unwired) TRUE
          # "radius"
          # "stretch"
          # "Nao precisa recalcular trajetória!\nEntao mantém a da iteração anterior"
          n97 = Multiply(x=-0.5, y=w376) -> (x*y=w380:dbl)
          n98 = Unbundle By Name(w375) -> ("x"=w385:dbl, "y"=w381:dbl, "function"=w387:T3)
          n99 = Add(x=w377, y=w380) -> (x+y=w379:dbl)
          n100 = Equal?(x=w387, y=Functions_Enum."Defender") -> ()  [unwired: 1 out]
          n101 = Index Array(array=w373) -> (element #1=w383:dbl, element #2=w382:dbl)  [unwired: 2 in]
          n102 = Index Array(array=w374) -> (element #1=w365:dbl, element #2=w371:dbl)  [unwired: 2 in]
          n103 = Subtract(x=w365, y=w383) -> (x-y=w369:dbl)
          n104 = Subtract(x=w371, y=w382) -> (x-y=w363:dbl)
          n105 = Build Array(w385, w381) -> (w367:dbl[])
          n106 = Absolute Value(x=w363) -> (abs(x)=w364:dbl)
          n107 = Greater Than 0?(x=w369) -> (x > 0?=w370:bool)
          n108 = Greater?(x=w364, y=w378) -> (0:w366:bool)
          n109 = case shown="True" w366 {
            tunnel: w370 -> [w394 _]
            tunnel: w369 -> [w393 _]
            tunnel: "Path out" -> [w392 w429]
            tunnel: [w391 w430] -> w372
            tunnel: w367 -> [w390 w427]
            tunnel: w373 -> [w389 w428]
            tunnel: w363 -> [w388 w423]
            tunnel: w379 -> [_ w420]
            tunnel: w365 -> [_ _]
            tunnel: w365 -> [_ w419]
            tunnel: w383 -> [_ w417]
            frame False {
              n110 = case shown="False" w394 {
                tunnel: w393 -> [w402 w413]
                tunnel: w388 -> [w404 w415]
                tunnel: w392 -> [w405 w416]
                tunnel: [w401 w412] -> w391
                tunnel: w390 -> [w400 w411]
                tunnel: w389 -> [w395 w406]
                frame True {
                  w403 = 0.0 ("element")
                  n111 = Build Array(w403, w404) -> (w398:dbl[])
                  n112 = Build Array(w402, w403) -> (w399:dbl[])
                  n113 = Add(x=w399, y=w400) -> (x+y=w396:dbl[])
                  n114 = Add(x=w396, y=w398) -> (x+y=w397:dbl[])
                  n115 = Insert Into Array(array=w405, new element #1=w395, new element #2=w396, new element #3=w397) -> (w401:dbl[][])  [unwired: 2 in]
                }
                frame False {
                  w414 = 0.0 ("element")
                  n116 = Build Array(w414, w415) -> (w410:dbl[])
                  n117 = Build Array(w413, w414) -> (w408:dbl[])
                  n118 = Add(x=w410, y=w411) -> (x+y=w409:dbl[])
                  n119 = Add(x=w409, y=w408) -> (x+y=w407:dbl[])
                  n120 = Insert Into Array(array=w416, new element #1=w406, new element #2=w409, new element #3=w407) -> (w412:dbl[][])  [unwired: 2 in]
                }
              }
            }
            frame True {
              w422 = 0.0 ("element")
              n121 = Subtract(x=w420, y=w417) -> (x-y=w421:dbl)
              n122 = Subtract(x=w419, y=w420) -> (x-y=w418:dbl)
              n123 = Build Array(w421, w422) -> (w433:dbl[])
              n124 = Build Array(w422, w423) -> (w431:dbl[])
              n125 = Build Array(w418, w422) -> (w425:dbl[])
              n126 = Add(x=w433, y=w427) -> (x+y=w432:dbl[])
              n127 = Add(x=w432, y=w431) -> (x+y=w426:dbl[])
              n128 = Add(x=w426, y=w425) -> (x+y=w424:dbl[])
              n129 = Insert Into Array(array=w429, new element #1=w428, new element #2=w432, new element #3=w426, new element #4=w424) -> (w430:dbl[][])  [unwired: 2 in]
            }
          }
          "Path out 2" <- w372
        }
      }
    }
  }
  "Path" <- w54
  n130 = Index Array(array=w67) -> (element=w58:T8)  [unwired: 1 in]
  n131 = call "SmoothPath.vi"("ignoreBall?"=w6, "ball"=w58, "defesa"=w51, "Initial State"="Initial Pos x,y", "Robot in"="Robot", "our_robots"=w60, "enemy_robots"=w59, "Path"=w54, "Goal"="Dest x,y") -> ("SmoothPath"=w57:dbl[][])  [unwired: 2 in]
  n132 = case shown="False" TRUE {
    tunnel: [w440 w441] -> w61
    tunnel: w60 -> [w439 _]
    tunnel: w59 -> [w438 _]
    tunnel: w58 -> [w437 _]
    tunnel: "Robot" -> [w436 _]
    tunnel: w57 -> [w435 w441]
    tunnel: w6 -> [w434 _]
    frame False {
      n133 = call "SmootherPath.vi"("ignoreBall?"=w434, "ball"=w437, "Robot in"=w436, "SmoothPath"=w435, "enemy_robots"=w438, "our_robots"=w439) -> ("SmootherPath"=w440:dbl[][])  [unwired: 5 in]
    }
    frame True {
    }
  }
  n134 = call "PrunePath.vi"("Robot in"="Robot", "Path in"=w61) -> ("Path out"=w53:dbl[][])  [unwired: 8 in, 1 out]
  "Smooth Path" <- w53
  n135 = feedback-in #1(w53) -> ()
